vi "keithley_6510_temperature_continuous_reading1.vi"() -> ()   [LabVIEW 2019]
panel:
  out "Waveform Graph":dbl[](graph)
  out "read buffer 2":string
  out "read buffer":string
  in  "stop":bool
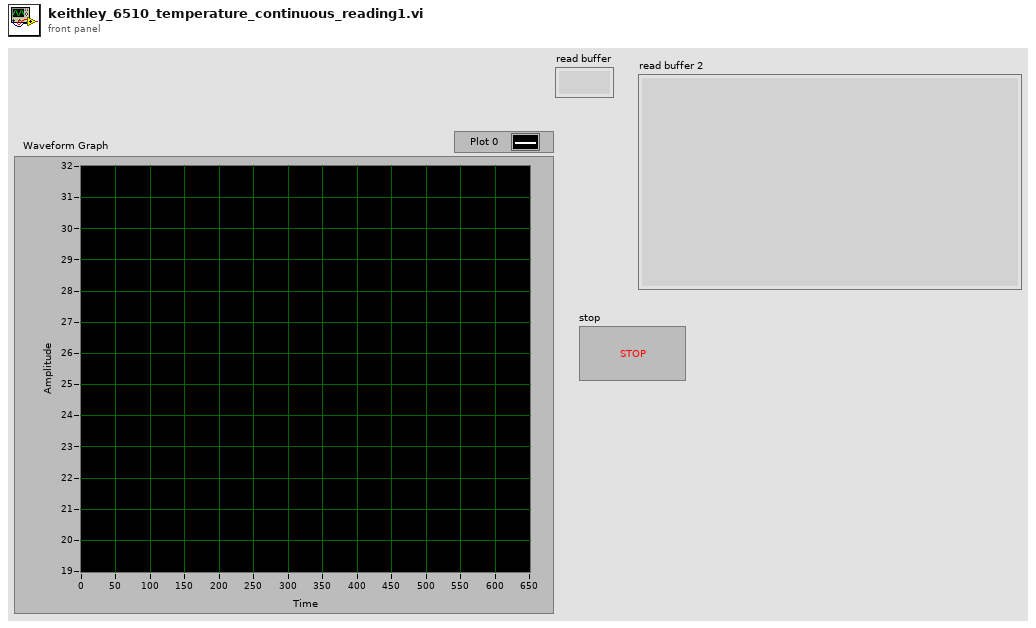
[diagram p1: front panel]
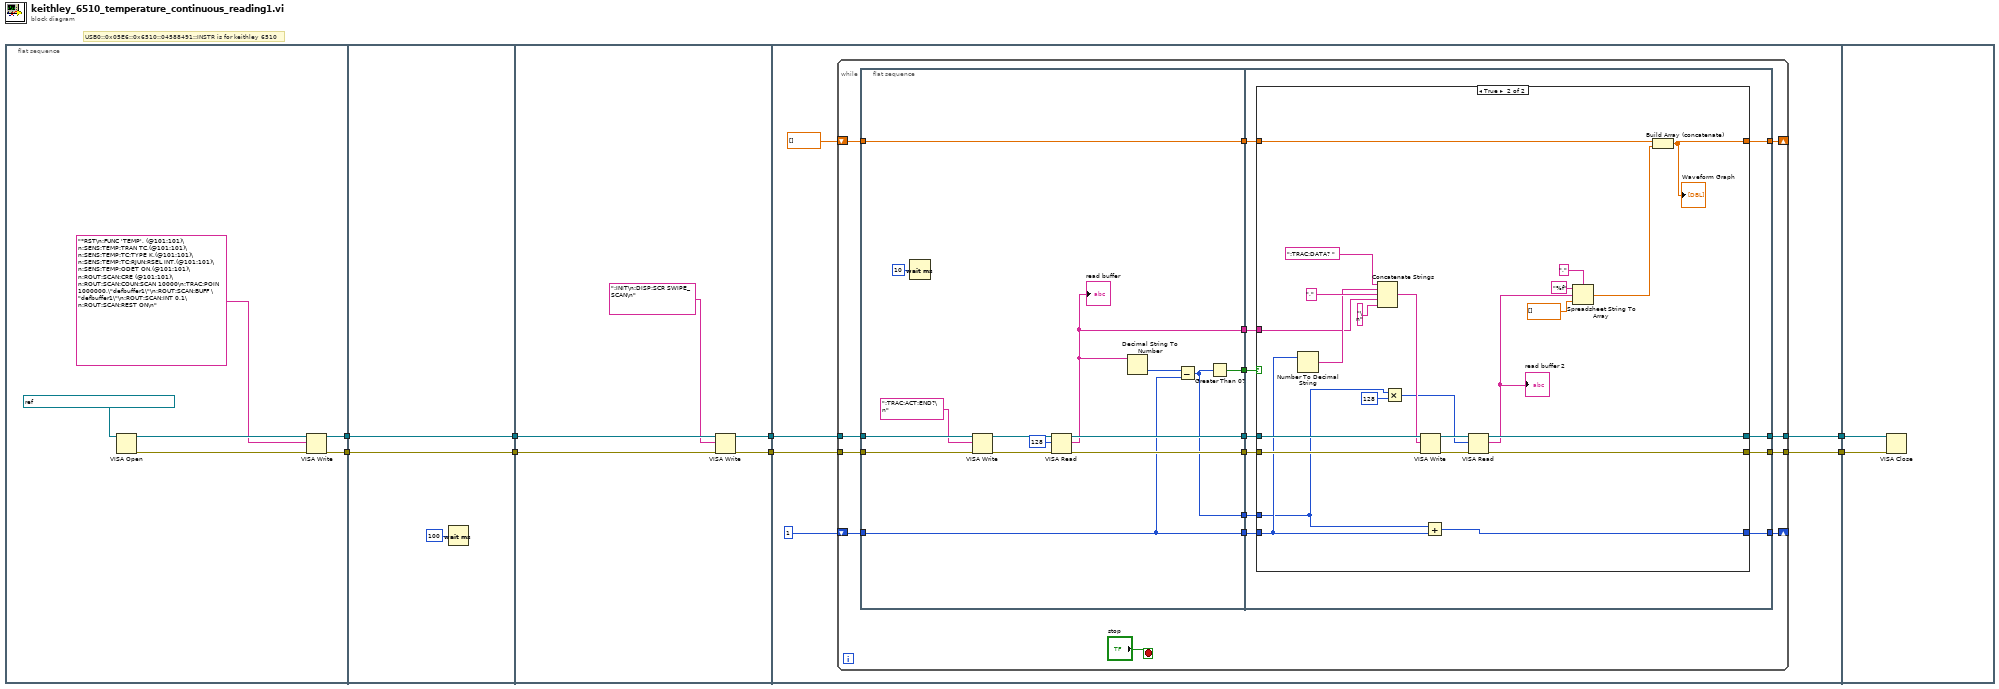
[diagram p0: block diagram]
diagram:
  # "USB0::0x05E6::0x6510::04588491::INSTR is for keithley 6510"
  n1 = flat-sequence {
    tunnel: [w11] -> w8
    tunnel: [w10] -> w7
    tunnel: w8 -> [w16]
    tunnel: w7 -> [w15]
    tunnel: [w16] -> w6
    tunnel: [w15] -> w5
    tunnel: w6 -> [w22]
    tunnel: w5 -> [w21]
    tunnel: [w19] -> w4
    tunnel: [w18] -> w3
    tunnel: w4 -> [w28]
    tunnel: w3 -> [w27]
    tunnel: [w26] -> w2
    tunnel: [w25] -> w1
    tunnel: w2 -> [w100]
    tunnel: w1 -> [w99]
    frame #0 {
      n2 = VISA Open(VISA resource name=refnum<visa-resource-name> "USB0::0x05E6::0x6510::04588491::INSTR") -> (VISA resource name=w13:refnum<visa-resource-name>, error out=w12:errorcluster)  [unwired: 4 in]
      n3 = VISA Write(VISA resource name=w13, write buffer="*RST\n:FUNC 'TEMP', (@101:101)\n:SENS:TEMP:TRAN TC,(@101:101)\n:SENS:TEMP:TC:TYPE K,(@101:101)\n:SENS:TEMP:TC:RJUN:RSEL INT,(@101:101)\n:SENS:TEMP:ODET ON,(@101:101)\n:ROUT:SCAN:CRE (@101:101)\n:ROUT:SCAN:COUN:SCAN 10000\n:TRAC:POIN 1000000,\"defbuffer1\"\n:ROUT:SCAN:BUFF \"defbuffer1\"\n:ROUT:SCAN:INT 0.1\n:ROUT:SCAN:REST ON\n", error in (no error)=w12) -> (VISA resource name out=w11:refnum<visa-resource-name>, error out=w10:errorcluster)  [unwired: 1 out]
    }
    frame #1 {
      n4 = Wait (ms)(milliseconds to wait=u32 100) -> ()  [unwired: 1 out]
    }
    frame #2 {
      n5 = VISA Write(VISA resource name=w22, write buffer=":INIT\n:DISP:SCR SWIPE_SCAN\n", error in (no error)=w21) -> (VISA resource name out=w19:refnum<visa-resource-name>, error out=w18:errorcluster)  [unwired: 1 out]
    }
    frame #3 {
      n6 = while {
        tunnel: w28 -> [w43]
        tunnel: w27 -> [w42]
        tunnel: [w41] -> w26
        tunnel: [w40] -> w25
        shift-right: [w34] -> _
        shift-left: 1 -> [w36]
        shift-right: [w29] -> _
        shift-left: dbl[] [] ("array type (2D Dbl)") -> [w31]
        stop <- "stop" stop-if-true
        n7 = flat-sequence {
          tunnel: w43 -> [w59]
          tunnel: w42 -> [w58]
          tunnel: [w54] -> w39
          tunnel: [w53] -> w38
          tunnel: [w50] -> w37
          tunnel: w36 -> [w47]
          tunnel: [w47] -> w35
          tunnel: [w49] -> w33
          tunnel: [w46] -> w32
          tunnel: w31 -> [w45]
          tunnel: [w45] -> w30
          tunnel: [w67] -> w40
          tunnel: [w68] -> w41
          tunnel: w39 -> [w70]
          tunnel: w38 -> [w69]
          tunnel: w37 -> [w66]
          tunnel: w35 -> [w65]
          tunnel: [w64] -> w34
          tunnel: w33 -> [w63]
          tunnel: w32 -> [w62]
          tunnel: w30 -> [w61]
          tunnel: [w60] -> w29
          frame #0 {
            n8 = Wait (ms)(milliseconds to wait=u32 10) -> ()  [unwired: 1 out]
            n9 = VISA Write(VISA resource name=w59, write buffer=":TRAC:ACT:END?\n", error in (no error)=w58) -> (VISA resource name out=w57:refnum<visa-resource-name>, error out=w56:errorcluster)  [unwired: 1 out]
            n10 = VISA Read(VISA resource name=w57, byte count=u32 128, error in (no error)=w56) -> (VISA resource name out=w54:refnum<visa-resource-name>, read buffer=w49:string, error out=w53:errorcluster)  [unwired: 1 out]
            "read buffer" <- w49
            n11 = Decimal String To Number(string=w49) -> (number=w48:i32)  [unwired: 2 in, 1 out]
            n12 = Subtract(x=w48, y=w47) -> (x-y=w46:i32)
            n13 = Greater Than 0?(x=w46) -> (x > 0?=w50:bool)
          }
          frame #1 {
            n14 = case shown="True" w66 {
              tunnel: w70 -> [w74 w96]
              tunnel: w69 -> [w73 w95]
              tunnel: [w74 w91] -> w68
              tunnel: [w73 w90] -> w67
              tunnel: w65 -> [w72 w88]
              tunnel: [w72 w86] -> w64
              tunnel: w63 -> [_ w85]
              tunnel: w62 -> [_ w83]
              tunnel: w61 -> [w71 w77]
              tunnel: [w71 w75] -> w60
              frame False {
              }
              frame True {
                n15 = Number To Decimal String(number=w88) -> (decimal integer string=w87:string)  [unwired: 1 in]
                n16 = Concatenate Strings(":TRAC:DATA? " ("string"), w87, "," ("string"), w85, "\n" ("string")) -> (w94:string)
                n17 = Multiply(x=w83, y=128) -> (x*y=w82:i32)
                n18 = VISA Write(VISA resource name=w96, write buffer=w94, error in (no error)=w95) -> (VISA resource name out=w93:refnum<visa-resource-name>, error out=w92:errorcluster)  [unwired: 1 out]
                n19 = Add(x=w83, y=w88) -> (x+y=w86:i32)
                n20 = VISA Read(VISA resource name=w93, byte count=w82, error in (no error)=w92) -> (VISA resource name out=w91:refnum<visa-resource-name>, read buffer=w78:string, error out=w90:errorcluster)  [unwired: 1 out]
                "read buffer 2" <- w78
                n21 = Spreadsheet String To Array(delimiter (Tab)=",", format string="%f", spreadsheet string=w78, array type (2D Dbl)=dbl[] []) -> (array=w76:dbl[])
                n22 = Build Array (concatenate)(w77, w76) -> (w75:dbl[])
                "Waveform Graph" <- w75
              }
            }
          }
        }
      }
    }
    frame #4 {
      n23 = VISA Close(VISA resource name=w100, error in (no error)=w99) -> ()  [unwired: 1 out]
    }
  }
